vi "replaceNameAndDateTokens.vi"(8 "error in (no error)":errorcluster, 10 "Querry In":string, 11 "Goal in":refnum<class "Goal.lvclass">) -> (0 "error out":errorcluster, 2 "Query Out":string, 3 "Goal out":refnum<class "Goal.lvclass">)   [LabVIEW 2018, in "Goal.lvclass"]
uses:
  Goal.lvclass
  Goal.lvclass/Goal.ctl
  WhichMonth/WhichMonth.lvclass
  Category/Category.lvclass
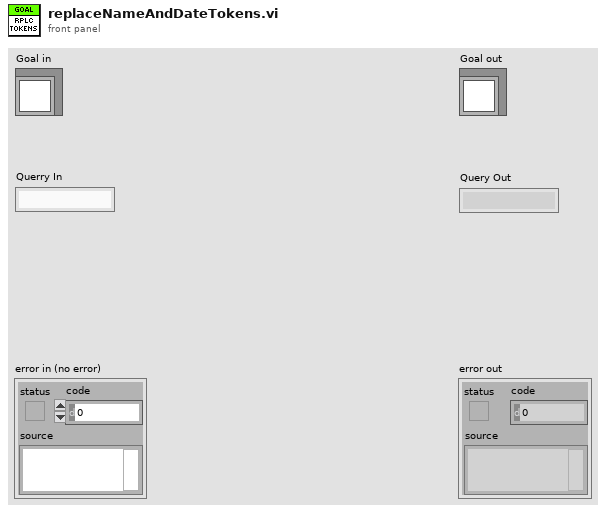
[diagram p1: front panel]
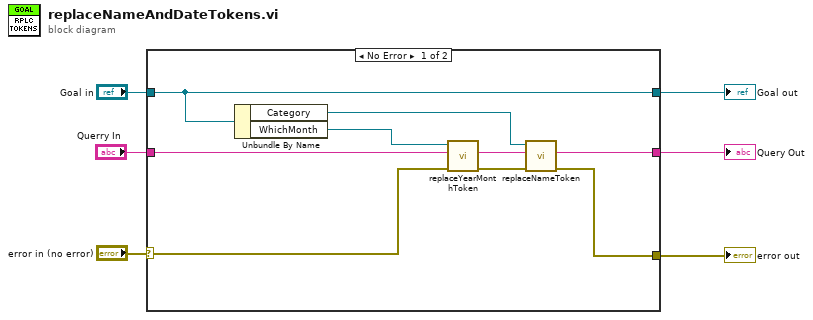
[diagram p0: block diagram]
diagram:
  n1 = case shown="No Error" "error in (no error)" {
    selector: "error in (no error)" -> [w13 w17]
    tunnel: [w7 w17] -> w5
    tunnel: [w15 w16] -> w3
    tunnel: "Goal in" -> [w15 w16]
    tunnel: [w8 _] -> w2
    tunnel: "Querry In" -> [w14 _]
    frame No Error {
      n2 = Unbundle By Name(w15) -> ("Category"=w11:refnum<class "Category.lvclass">, "WhichMonth"=w12:refnum<class "WhichMonth.lvclass">)
      n3 = call "replaceYearMonthToken.vi"("error in (no error)"=w13, "Query In"=w14, "WhichMonth in"=w12) -> ("error out"=w9:errorcluster, "Query Out"=w10:string)  [unwired: 6 in, 1 out]
      n4 = call "replaceNameToken.vi"("error in (no error)"=w9, "Query In"=w10, "Category in"=w11) -> ("error out"=w7:errorcluster, "Query Out"=w8:string)  [unwired: 6 in, 1 out]
    }
    frame Error {
    }
  }
  "error out" <- w5
  "Goal out" <- w3
  "Query Out" <- w2
